vi "LVClasse_HasoConfig Write HasoConfig.vi"(8 "error in (no error)":errorcluster, 10 "Surface":i32, 11 "Surface in":refnum<class "HasoConfig.lvclass">) -> (0 "error out":errorcluster, 3 "Surface out":refnum<class "HasoConfig.lvclass">)   [LabVIEW 2020, in "HasoConfig.lvclass"]
uses:
  HasoConfig.lvclass
  HasoConfig.lvclass/HasoConfig.ctl
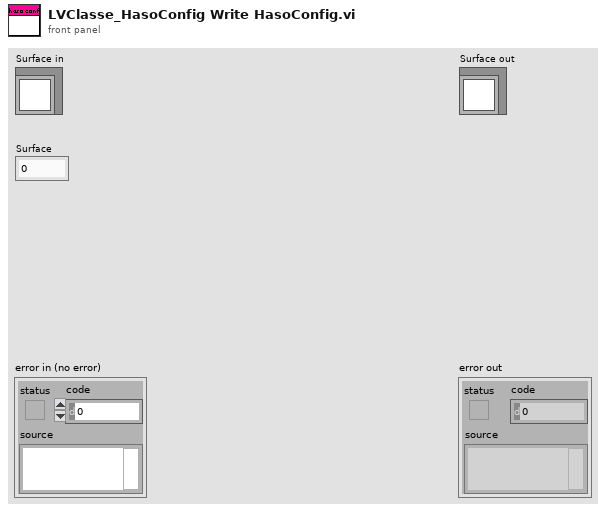
[diagram p1: front panel]
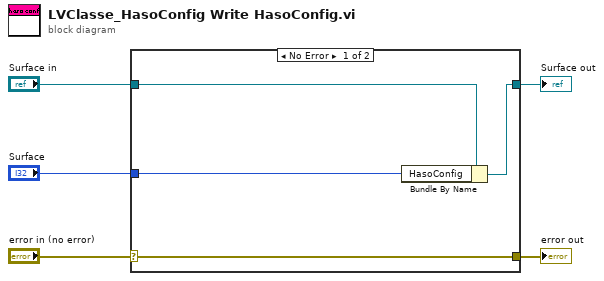
[diagram p0: block diagram]
diagram:
  n1 = case shown="No Error" "error in (no error)" {
    selector: "error in (no error)" -> [w9 w10]
    tunnel: [w9 w10] -> w4
    tunnel: [w7 w11] -> w2
    tunnel: "Surface in" -> [w8 w11]
    tunnel: "Surface" -> [w6 _]
    frame No Error {
      n2 = Bundle By Name(cluster=w8, "HasoConfig"=w6) -> (w7:refnum<class "HasoConfig.lvclass">)
    }
    frame Error {
    }
  }
  "error out" <- w4
  "Surface out" <- w2
